vi "play_TEST_LoadObserverControlMatrix_MIMO_MPC.vi"() -> ()   [LabVIEW 2017]
uses:
  <vilib>/rvi/interface/nirviMethod/nirviMethod.xnode
  <vilib>/rvi/errors/niLvFpgaMergeErrorWithErrorCode.vi
  <vilib>/rvi/interface/nirviReadWriteControl/nirviReadWriteControl.xnode
  <vilib>/rvi/errors/niLvFpgaAdjustHostInterfaceError.vi
  <vilib>/rvi/interface/nirviOpenFPGA/nirviOpenFPGA.xnode
  <vilib>/userdefined/High Color/nirio_resource_hc.ctl
  <vilib>/FPGAPlugInAG/Dynamic/niLvFpga_Reset_Dynamic.vi
  <vilib>/rvi/interface/Simulation/niFpgaSimulationCallBeginRW.vi
  <vilib>/FPGAPlugInAG/Dynamic/niLvFpga_Run_Dynamic.vi
  FPGA Bitfiles/afmMPCmultiAxis_FPGATarget_TESTLoadObserver_MPC.lvbitx
  <vilib>/FPGAPlugInAG/Dynamic/niLvFpga_ConfigureFifo_Dynamic.vi
  <vilib>/FPGAPlugInAG/Dynamic/niLvFpga_WriteFifo_Dynamic.vi
  <vilib>/FPGAPlugInAG/cRIO-9082/niLvFpga_Open_cRIO-9082.vi
  <vilib>/rvi/interface/common/dynamic/niFpgaDynamicAddResources.vi
  fpga_VIs/fixed-point/typeDefs/FXPControlParams_distEst.ctl
  fpga_VIs/fixed-point/single-axis/fxp_mpc/fgm_pipiline/quadProgParams_pipe.ctl
  controls/ObserverMatrices.ctl
panel:
  out "ControlMatrices":T1
  out "QP_params":T2={"maxIter"=0, "nuN"=24, "Ns_mpc"=0, "-beta"=-0.9987945556640625, "beta+1"=1.9987945556640625}
  in  "Tab Control":enum32{"Page 1", "Page 2"}(tab)
  out "MPC matrices":dbl[][](array[numeric])
  in  "Mem Select":T3(ring)
  out "mpcRowHost":dbl[](array[numeric])
  in  "mpcRowHost":i32
  out "Data Out":fxp<+/-,32,8>[](array[numeric])
  out "ControlParamsMpc 2":T4={"umax"=3.0, "NS"=0, "ref_f_VEC"=[0.0, 0.0], "du_max"=0.0}
  out "Ns":u16
  in  "RowStart*Ns":u16
  out "Data Out cpy":fxp<+/-,32,3>[](array[numeric])
  in  "stop":bool
  out "Empty Elements Remaining":u32
  in  "control_data_path":path=path "C:/Users/arnold/Documents/MATLAB/AFM_MPC/data/exp_multiAxis.csv"
  out "y iter":i32
  # "NOTE: Ns is the number of states in the plant. The number of states in the \nobserver is Ns+1. Thus, for B, L, C, and A, we use NS+1. For K and Xss, we use Ns\nbecause the controller does not operate on the disturbance state, Xd."
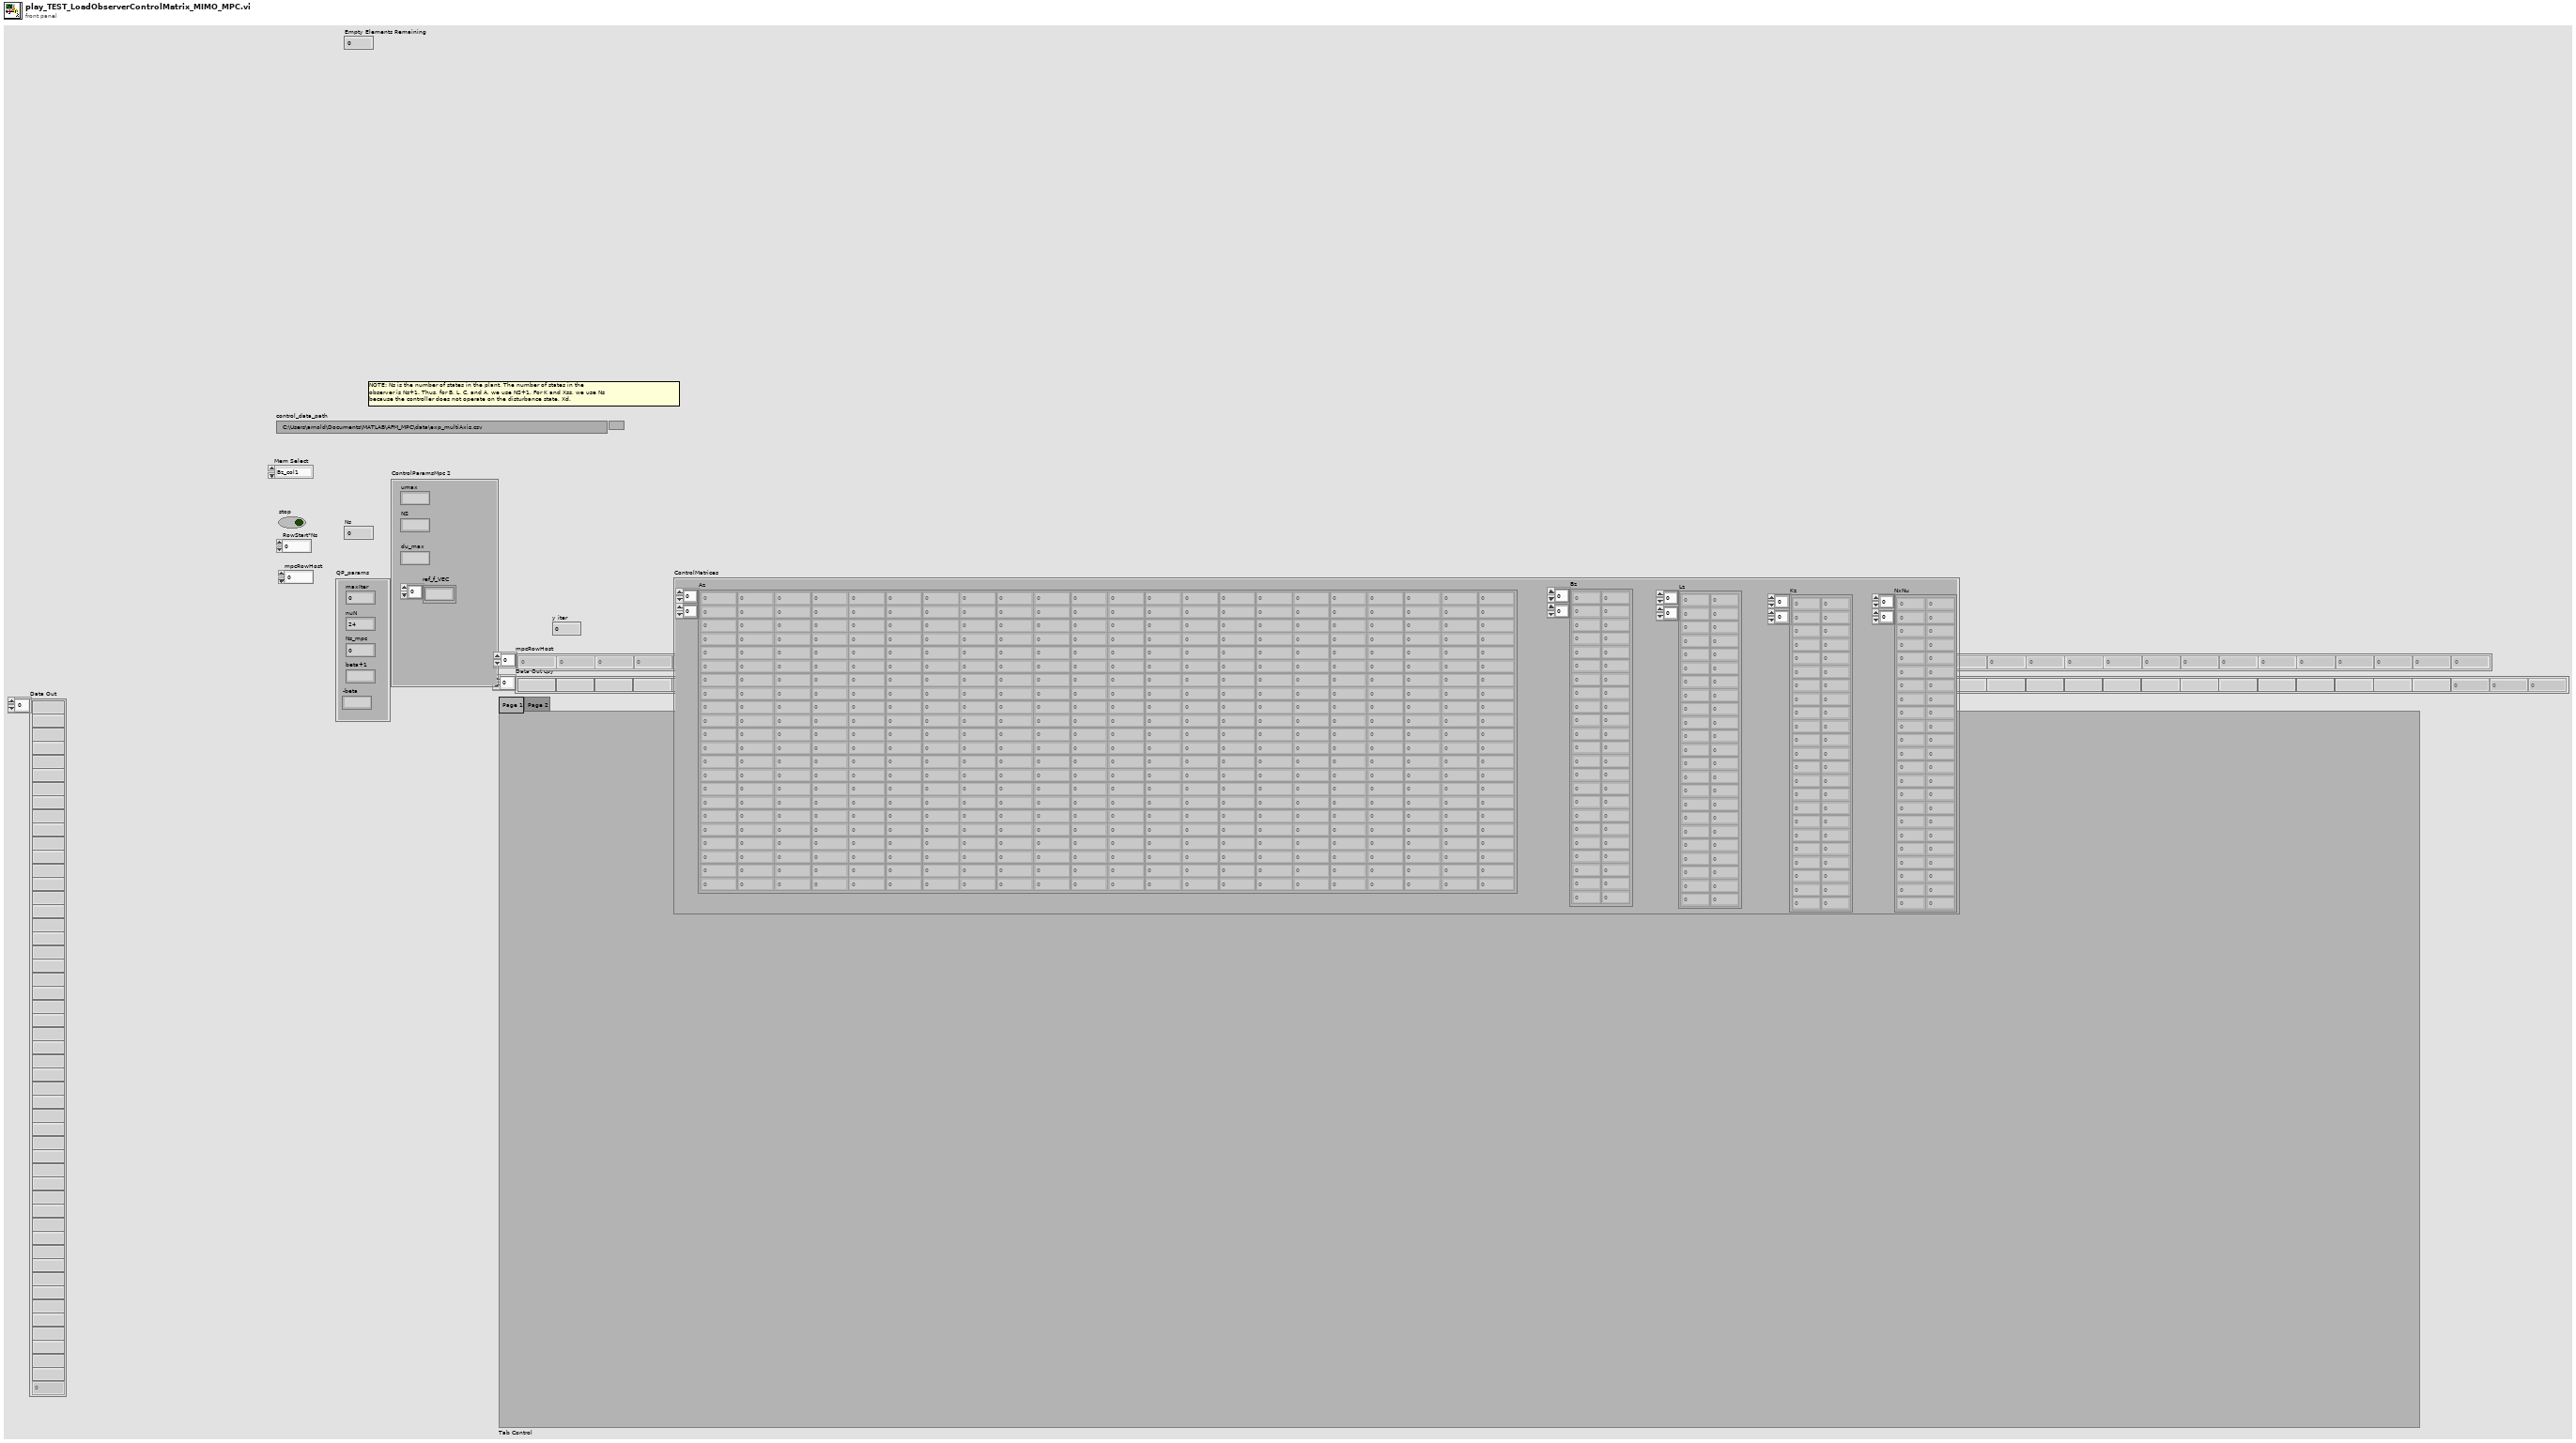
[diagram p1: front panel]
types:
  T1 = typedef "ObserverMatrices.ctl" = cluster{"Az":fxp<+/-,32,4>[][], "Bz":dbl[][], "Lz":dbl[][], "Kz":dbl[][], "NxNu":dbl[][]}
  T2 = typedef "quadProgParams_pipe.ctl" = cluster{"maxIter":u16, "nuN":u16, "Ns_mpc":u16, "-beta":fxp<+/-,18,2>, "beta+1":fxp<+/-,18,2>}
  T3 = enum16{"Bz_col1", "Bz_col2", "L_col1", "L_col2", "Az", "Nx_col1", "Nx_col2", "MPC1", "MPC2", "MPC3", "MPC4", "MPC5", "MPC6", "MPC7", "MPC8", "MPC9", "MPC10", "MPC11", "MPC12", "MPC13", "MPC14", "MPC15", "MPC16", "MPC17", "MPC18", "MPC19", "MPC20", "MPC21", "MPC22", "MPC23", "MPC24"}
  T4 = typedef "FXPControlParams_distEst.ctl" = cluster{"umax":fxp<+/-,18,5>, "NS":u8, "ref_f_VEC":fxp<+/-,32,5>[], "du_max":fxp<+/-,18,5>}
  T5 = typedef "nirio_resource_hc.ctl" = tag
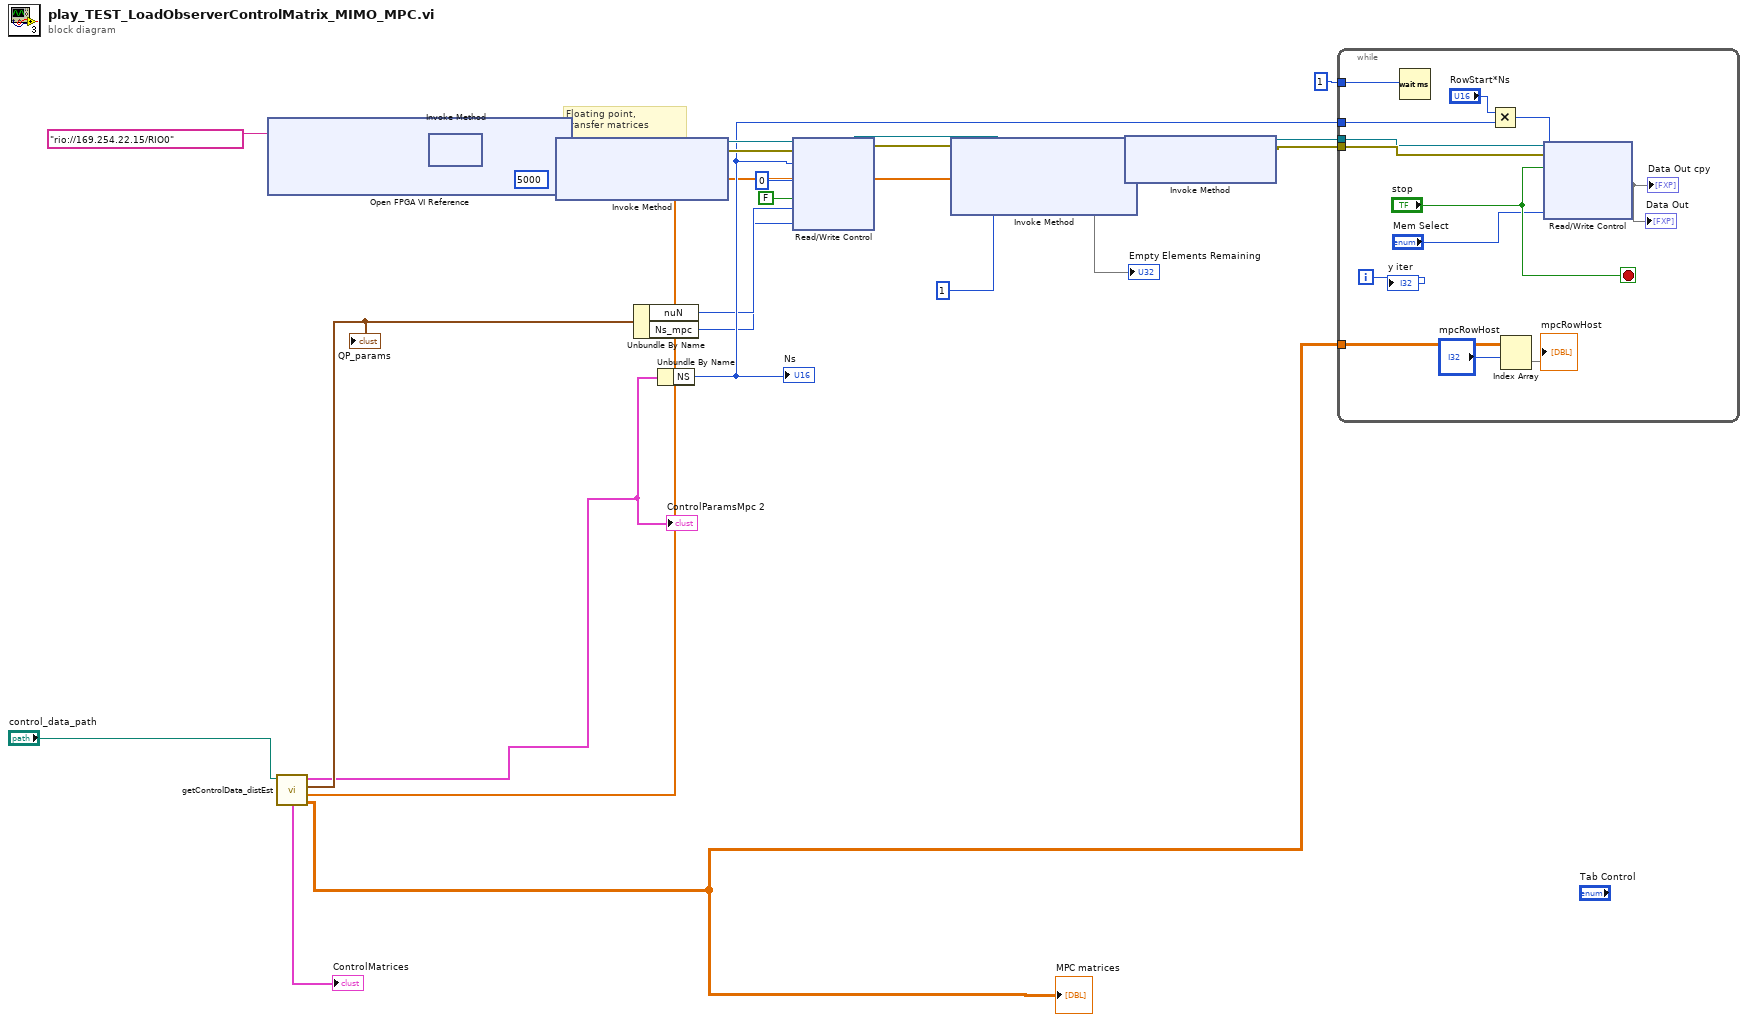
[diagram p0: block diagram]
diagram:
  # "Floating point, \ntransfer matrices"
  n1 = xnode "Open FPGA VI Reference"("resource name"=T5 "rio://169.254.22.15/RIO0") -> ("FPGA VI Reference Out"=w21:refnum<k20>, "error out"=w23:errorcluster)  [unwired: 1 in]
  n2 = call "getControlData_distEst.vi"("system matricec path"="control_data_path") -> ("MPC matrices"=w1:dbl[][], "AllMatrix"=w3:dbl[], "QP_params"=w6:T2, "ControlParams"=w5:T4, "ControlMatrices"=→"ControlMatrices":T1)  [unwired: 6 in]
  "ControlParamsMpc 2" <- w5
  "MPC matrices" <- w1
  "QP_params" <- w6
  n3 = xnode "Invoke Method"("FPGA VI Reference In"=w21, "error in"=w23) -> ("FPGA VI Reference Out"=w20:refnum<k20>, "error out"=w19:errorcluster)
  n4 = xnode "Invoke Method"("FPGA VI Reference In"=w20, "error in"=w19, "Requested Depth"=u32 5000) -> ("FPGA VI Reference Out"=w14:refnum<k20>, "error out"=w13:errorcluster)  [unwired: 1 out]
  n5 = Unbundle By Name(w6) -> ("nuN"=w9:u16, "Ns_mpc"=w8:u16)
  n6 = Unbundle By Name(w5) -> ("NS"=w10:u8)
  "Ns" <- w10
  n7 = xnode "Read/Write Control"("FPGA VI Reference In"=w14, "error in"=w13, "Ns"=w10, "Row start"=u16 0 ("RowToRead"), "stop"=FALSE, "nuN"=w9, "Row start"=w8) -> ("FPGA VI Reference Out"=w25:refnum<k20>, "error out"=w24:errorcluster)
  n8 = xnode "Invoke Method"("FPGA VI Reference In"=w25, "error in"=w24, "Data"=w3, "Timeout (ms)"=1) -> ("FPGA VI Reference Out"=w27:refnum<k20>, "error out"=w26:errorcluster, "Empty Elements Remaining"=→"Empty Elements Remaining")
  n9 = xnode "Invoke Method"("FPGA VI Reference In"=w27, "error in"=w26) -> ("FPGA VI Reference Out"=w16:refnum<k20>, "error out"=w15:errorcluster)  [unwired: 1 in]
  n10 = while {
    tunnel: 1 -> [w41]
    tunnel: w16 -> [w39]
    tunnel: w15 -> [w40]
    tunnel: w10 -> [w33]
    tunnel: w1 -> [w32]
    i -> [w38]
    stop <- "stop" stop-if-true
    n11 = Wait (ms)(milliseconds to wait=w41) -> ()  [unwired: 1 out]
    n12 = Multiply(x="RowStart*Ns", y=w33) -> (x*y=w35:u16)
    n13 = Index Array(array=w32, index (row)="mpcRowHost") -> (element=→"mpcRowHost":dbl[])  [unwired: 1 in]
    n14 = xnode "Read/Write Control"("FPGA VI Reference In"=w39, "error in"=w40, "stop"="stop", "Row start"=w35, "Mem Select"="Mem Select") -> ("Array"=→"Data Out cpy" →"Data Out")  [unwired: 2 out]
    "y iter" <- w38
  }
